vi "Insert Transfer Data into Group.vi"(5 "transfer id":i32, 7 "transfer group id":i32, 8 "error in (no error)":errorcluster, 9 "transfer data":string, 10 "group data in":string, 11 "UDP Transceiver in":refnum<class "DSF UDP Transceiver.lvclass">) -> (0 "error out":errorcluster, 2 "group data out":string, 3 "UDP Transceiver out":refnum<class "DSF UDP Transceiver.lvclass">)   [LabVIEW 2017, in "DSF Core.lvlib" / "DSF UDP Transceiver.lvclass"]
uses:
  DSF UDP Transceiver.lvclass
  DSF UDP Transceiver.lvclass/DSF UDP Transceiver.ctl
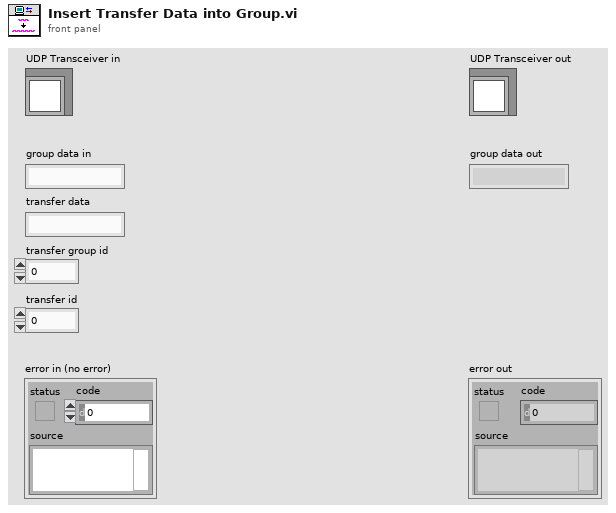
[diagram p1: front panel]
types:
  T1 = typedef "DSF Core.lvlib/DSF UDP Transceiver.lvclass/Transfer Group Parameters.ctl" = cluster{"transfers":T2[], "max size":i32, "timeout":i32}
  T2 = typedef "DSF Core.lvlib/DSF UDP Transceiver.lvclass/Transfer Parameters.ctl" = cluster{"group offset":u64, "size":u64, "address":u32, "port":u16}
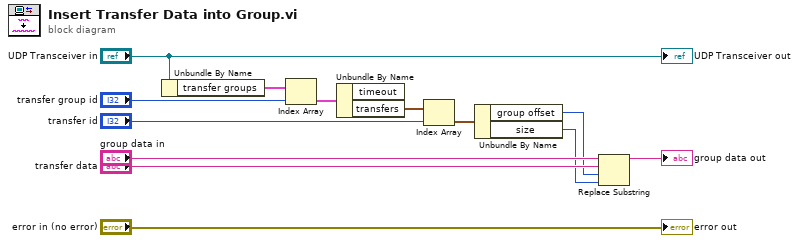
[diagram p0: block diagram]
diagram:
  n1 = Unbundle By Name("UDP Transceiver in") -> ("transfer groups"=w13:T1[])
  n2 = Index Array(array=w13, index="transfer group id") -> (element=w12:T1)
  n3 = Unbundle By Name(w12) -> ("transfers"=w10:T2[])  [unwired: 1 out]
  n4 = Index Array(array=w10, index="transfer id") -> (element=w11:T2)
  n5 = Unbundle By Name(w11) -> ("group offset"=w1:u64, "size"=w2:u64)
  n6 = Replace Substring(2:w2, 3:w1, 4:"transfer data", 5:"group data in") -> (1:→"group data out":string)  [unwired: 1 out]
  "error out" <- "error in (no error)"
  "UDP Transceiver out" <- "UDP Transceiver in"
